vi "flush.vi"(8 "error in (no error)":errorcluster, 10 "out?":bool, 11 "py in":T1) -> (0 "error out":errorcluster, 3 "py out":T1)   [LabVIEW 2022 SP3, in "pythonq.lvlib"]
uses:
  pythonq.lvlib
  py_session.ctl
  py_cluster.ctl
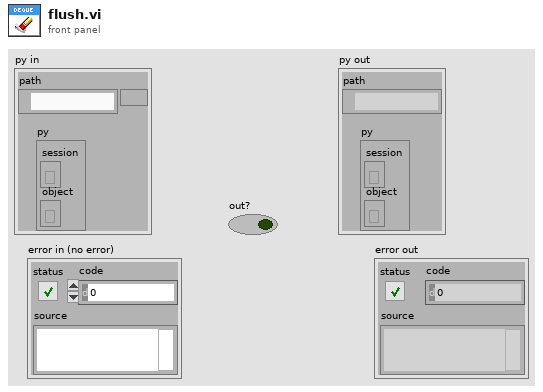
[diagram p1: front panel]
types:
  T1 = typedef "pythonq.lvlib/py_cluster.ctl" = cluster{"path":path, "py":T2}
  T2 = typedef "pythonq.lvlib/py_session.ctl" = cluster{"session":refnum<k35>, "object":refnum<k38>}
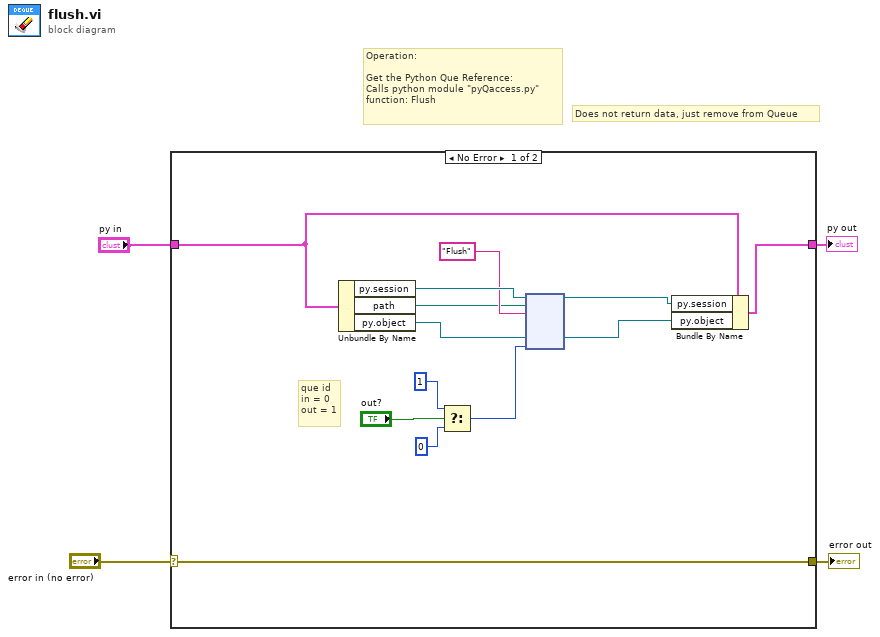
[diagram p0: block diagram]
diagram:
  # "Does not return data, just remove from Queue"
  # "Operation:\n\nGet the Python Que Reference:\nCalls python module \"pyQaccess.py\"\nfunction: Flush"
  n1 = case shown="No Error" "error in (no error)" {
    selector: "error in (no error)" -> [w17 w19]
    tunnel: "py in" -> [w7 w18]
    tunnel: [w6 w18] -> w3
    tunnel: [w17 w19] -> w1
    frame No Error {
      # "que id\nin = 0\nout = 1"
      n2 = Unbundle By Name(w7) -> ("py.session"=w15:refnum<k35>, "path"=w11:path, "py.object"=w16:refnum<k38>)
      n3 = Select(t=1, s="out?", f=0) -> (s? t:f=w8:i32)
      n4 = node(w15, w11, "Flush" ("function name"), w16, w8) -> (w13:refnum<k35>, w12:refnum<k38>)  [unwired: 4 in, 3 out]
      n5 = Bundle By Name(cluster=w7, "py.session"=w13, "py.object"=w12) -> (w6:T1)
    }
    frame Error {
    }
  }
  "error out" <- w1
  "py out" <- w3
